vi "CheckTimeSlot.vi"(0 "connection ID in":refnum<k5>, 1 "starttime":string, 2 "endtime":string, 3 "error in":errorcluster) -> (4 "Timeslot In Range?":bool, 5 "connection ID out":refnum<k5>, 6 "starttime out":string, 7 "endtime out":string, 8 "error out":errorcluster)   [LabVIEW 2010]
panel:
  out "date/time string":string
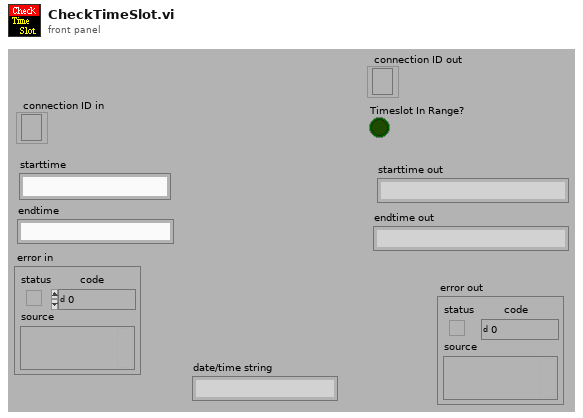
[diagram p1: front panel]
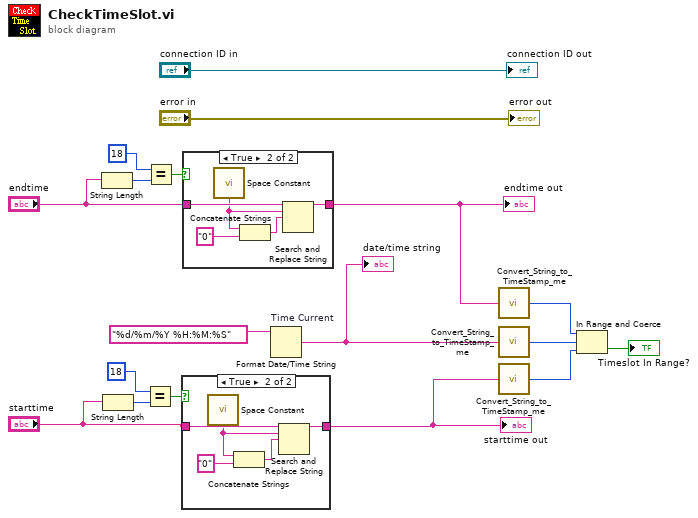
[diagram p0: block diagram]
diagram:
  n1 = String Length(string="endtime") -> (length=w13:i32)
  n2 = String Length(string="starttime") -> (length=w8:i32)
  n3 = Equal?(x=18, y=w8) -> (x = y?=w10:bool)
  n4 = Equal?(x=18, y=w13) -> (x = y?=w14:bool)
  n5 = case shown="True" w10 {
    tunnel: "starttime" -> [w19 w24]
    tunnel: [w19 w23] -> w2
    frame False {
    }
    frame True {
      n6 = call <vilib>:"Space Constant.vi"() -> ("String"=w20:string)
      n7 = Concatenate Strings(w20, "0" ("replace string (\"\")")) -> (w21:string)
      n8 = Search and Replace String(input string=w24, search string=w20, replace string=w21) -> (result string=w23:string)  [unwired: 1 in, 7 out]
    }
  }
  "starttime out" <- w2
  n9 = case shown="True" w14 {
    tunnel: "endtime" -> [w25 w30]
    tunnel: [w25 w29] -> w4
    frame False {
    }
    frame True {
      n10 = call <vilib>:"Space Constant.vi"() -> ("String"=w28:string)
      n11 = Concatenate Strings(w28, "0" ("replace string (\"\")")) -> (w26:string)
      n12 = Search and Replace String(input string=w30, search string=w28, replace string=w26) -> (result string=w29:string)  [unwired: 1 in, 7 out]
    }
  }
  "endtime out" <- w4
  n13 = Format Date/Time String "Time Current"(time format string (%c)="%d/%m/%Y %H:%M:%S") -> (date/time string=w6:string)  [unwired: 2 out]
  "date/time string" <- w6
  n14 = call "Convert_String_to_TimeStamp_me.vi"("string timestamp"=w4) -> ("seconds"=w3:u32)
  n15 = call "Convert_String_to_TimeStamp_me.vi"("string timestamp"=w6) -> ("seconds"=w5:u32)
  n16 = call "Convert_String_to_TimeStamp_me.vi"("string timestamp"=w2) -> ("seconds"=w1:u32)
  n17 = In Range and Coerce(upper limit=w3, x=w5, lower limit=w1) -> (In Range?=→"Timeslot In Range?":bool)  [unwired: 1 out]
  "connection ID out" <- "connection ID in"
  "error out" <- "error in"
